vi "ReadGPSInfo.vi"(0 "filepath":string, 1 "ExifTool Path":path=path "C:/Windows/System32", 11 "error in (no error)":errorcluster, 12 "wait until completion? (T)":bool=TRUE) -> (3 "Raw GPS Info":string, 4 "Version ID":string, 6 "Longitude":string, 8 "altitude":string, 10 "Latitude":string, 13 "standard error":string, 14 "Unknown":string, 15 "error out":errorcluster)   [LabVIEW 2016]
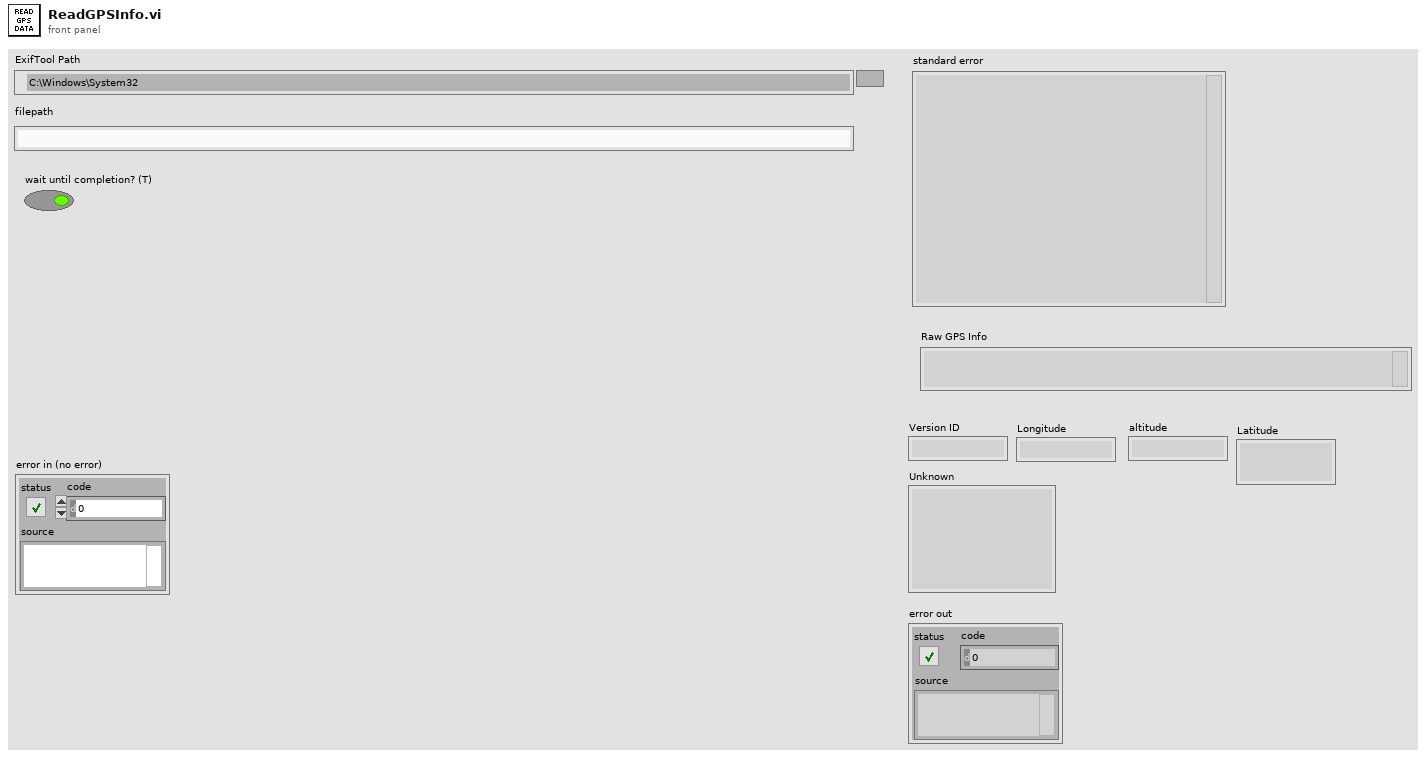
[diagram p1: front panel]
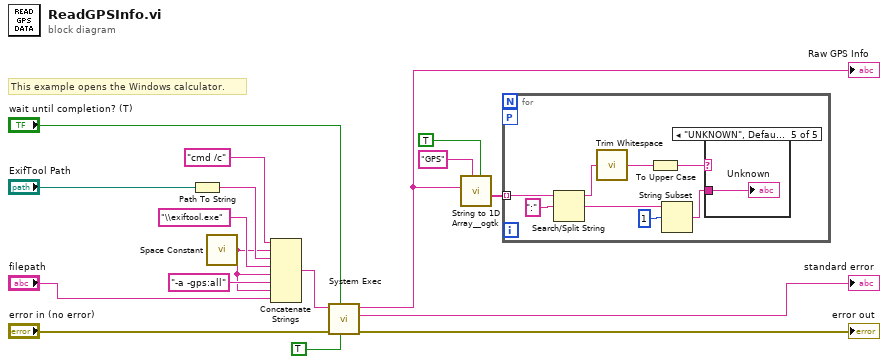
[diagram p0: block diagram]
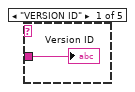
[diagram p2: hidden frame]
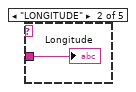
[diagram p3: hidden frame]
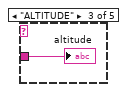
[diagram p4: hidden frame]
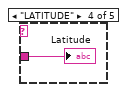
[diagram p5: hidden frame]
diagram:
  # "This example opens the Windows calculator."
  n1 = Path To String(path="ExifTool Path") -> (string=w14:string)
  n2 = call <vilib>:"Space Constant.vi"() -> ("String"=w6:string)
  n3 = Concatenate Strings("cmd /c" ("string"), w6, w14, "\\exiftool.exe" ("string"), w6, "-a -gps:all" ("string"), w6, "filepath") -> (w11:string)
  n4 = call <vilib>:"System Exec.vi"("run minimized? (F)"=TRUE, "wait until completion? (T)"="wait until completion? (T)", "error in (no error)"="error in (no error)", "command line"=w11) -> ("error out"=→"error out":errorcluster, "standard error"=→"standard error":string, "standard output"=w3:string)  [unwired: 4 in, 1 out]
  "Raw GPS Info" <- w3
  n5 = call <userlib>:"String to 1D Array__ogtk.vi"("ignore duplicate delimiters? (F=No)"=TRUE, "delimiter (Tab)"="GPS", "string"=w3) -> ("Array of Strings"=w1:string[])  [unwired: 8 in]
  n6 = for {
    tunnel: w1 -> [w25] mode=indexing
    workers-P: _ -> [_]
    n7 = Search/Split String(string=w25, search string/char (-)=":") -> (substring before match=w23:string, match + rest of string=w20:string)  [unwired: 1 in, 1 out]
    n8 = call <vilib>:"Trim Whitespace.vi"("string"=w23) -> ("trimmed string"=w22:string)  [unwired: 1 in]
    n9 = To Upper Case(1:w22) -> (0:w21:string)
    n10 = String Subset(string=w20, offset (0)=1) -> (substring=w18:string)  [unwired: 1 in]
    n11 = case shown="\"UNKNOWN\", Default" w21 {
      tunnel: w18 -> [w26 w27 w28 w29 w30]
      frame "VERSION ID" {
        "Version ID" <- w26
      }
      frame "LONGITUDE" {
        "Longitude" <- w27
      }
      frame "ALTITUDE" {
        "altitude" <- w28
      }
      frame "LATITUDE" {
        "Latitude" <- w29
      }
      frame "UNKNOWN", Default {
        "Unknown" <- w30
      }
    }
  }
